vi "LEP_RV_GenerateXMLFromLinkerMapFile.vi"(9 "Linker flags":string, 10 "Compiler flags":string, 11 "Project path":path) -> ()   [LabVIEW 2011]
panel:
  out "error out":errorcluster
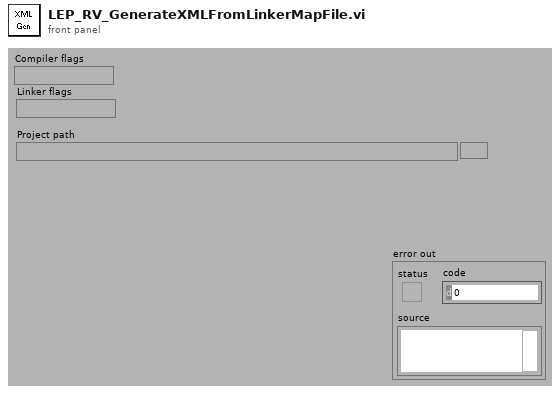
[diagram p1: front panel]
types:
  T1 = enum16{"open", "replace", "create", "open or create", "replace or create", "replace or create with confirmation"}
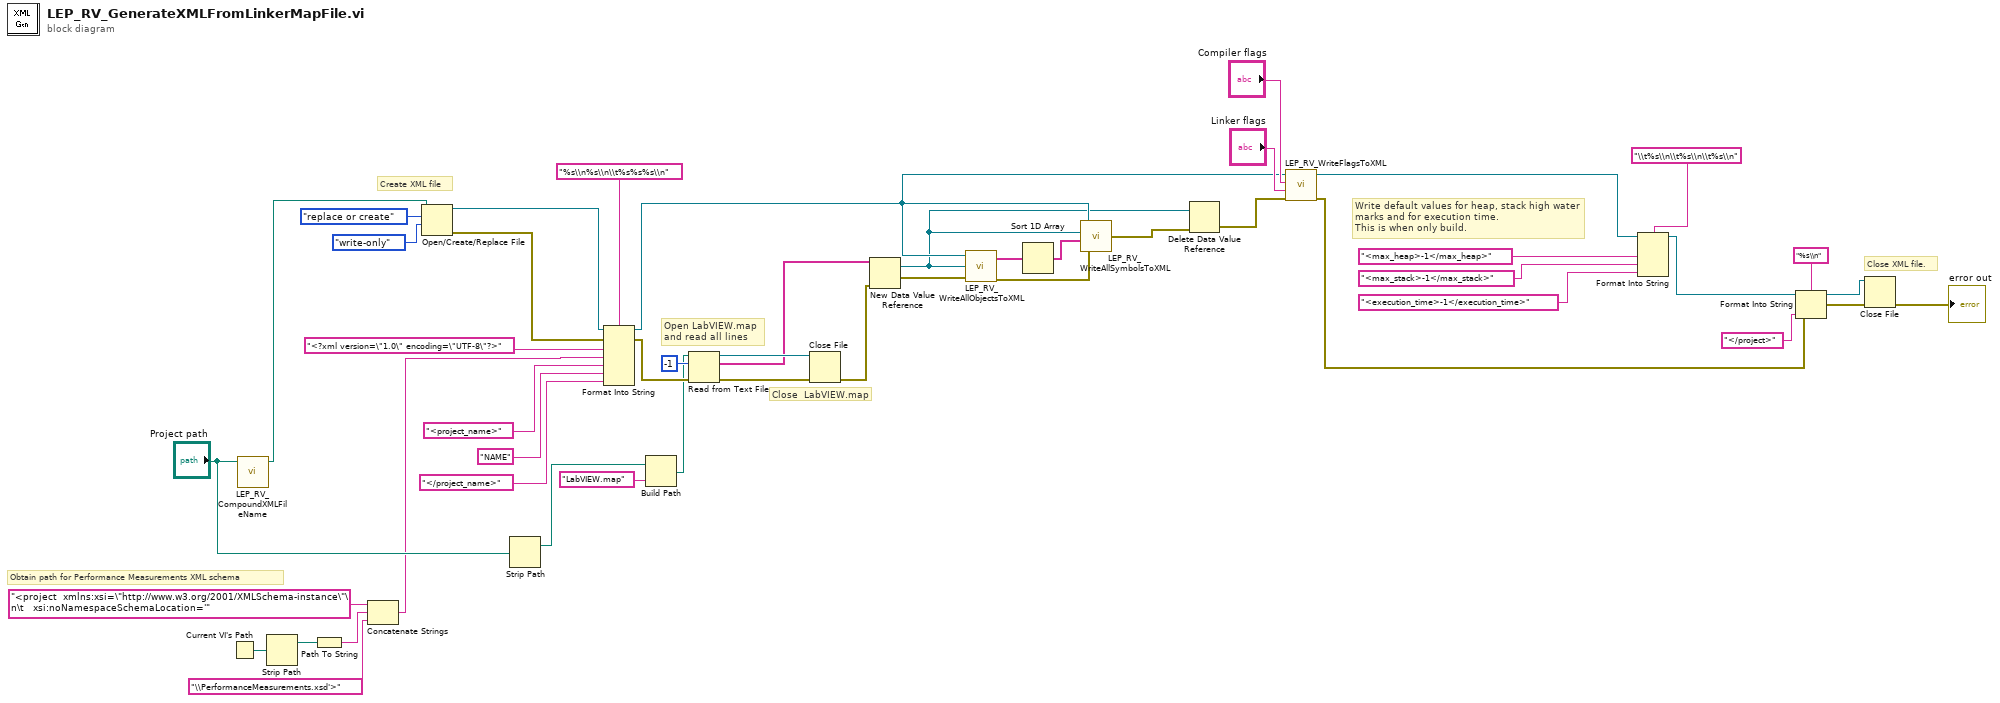
[diagram p0: block diagram]
diagram:
  # "Obtain path for Performance Measurements XML schema"
  # "Write default values for heap, stack high water marks and for execution time.\nThis is when only build."
  # "Close XML file."
  # "Close  LabVIEW.map"
  # "Open LabVIEW.map \nand read all lines"
  # "Create XML file"
  n1 = Current VI's Path() -> (path=w6:path)
  n2 = call "LEP_RV_CompoundXMLFileName.vi"("Project file path"="Project path") -> ("Path for XML generated file"=w19:path)  [unwired: 10 in]
  n3 = Strip Path(path=w6) -> (stripped path=w5:path)  [unwired: 1 out]
  n4 = Path To String(path=w5) -> (string=w3:string)
  n5 = Concatenate Strings("<project  xmlns:xsi=\"http://www.w3.org/2001/XMLSchema-instance\"\n\t   xsi:noNamespaceSchemaLocation='", w3, "\\PerformanceMeasurements.xsd'>") -> (w1:string)
  n6 = Open/Create/Replace File(file path (use dialog)=w19, operation (0:open)=T1."replace or create", access (0:read/write)=enum16{"read/write", "read-only", "write-only"}."write-only") -> (refnum out=w45:refnum<file>, error out=w44:errorcluster)  [unwired: 3 in, 1 out]
  n7 = Strip Path(path="Project path") -> (stripped path=w17:path)  [unwired: 1 out]
  n8 = Format Into String(format string="%s\\n%s\\n\\t%s%s%s\\n", initial string=w45, error in=w44, "<?xml version=\"1.0\" encoding=\"UTF-8\"?>" ("text"), w1, "<project_name>" ("input 3"), "NAME" ("input 4"), "</project_name>" ("input 5")) -> (resulting string=w21:refnum<file>, error out=w28:errorcluster)
  n9 = Build Path(base path=w17, name or relative path="LabVIEW.map") -> (appended path=w15:path)
  n10 = Read from Text File(file (use dialog)=w15, count=-1, error in=w28) -> (refnum out=w30:refnum<file>, text=w24:string[], error out=w29:errorcluster)  [unwired: 1 in, 1 out]
  n11 = Close File(refnum=w30, error in=w29) -> (error out=w23:errorcluster)  [unwired: 1 out]
  n12 = New Data Value Reference(data value=w24, error in=w23) -> (data value reference=w13:refnum<data-value>, error out=w22:errorcluster)
  n13 = call "LEP_RV_WriteAllObjectsToXML.vi"("error in"=w22, "Data value reference for\nLabVIEW.map file's lines array"=w13, "XML File Refnum"=w21) -> ("error out"=w25:errorcluster, "Array with objects' names"=w27:string[])
  n14 = Sort 1D Array(array=w27) -> (sorted array=w26:string[])
  n15 = call "LEP_RV_WriteAllSymbolsToXML.vi"("error in"=w25, "Sorted objects' names array"=w26, "Data value reference for\nLabVIEW.map file's lines array"=w13, "XML File Refnum"=w21) -> ("error out"=w14:errorcluster)
  n16 = Delete Data Value Reference(data value reference=w13, error in=w14) -> (error out=w20:errorcluster)  [unwired: 1 out]
  n17 = call "LEP_RV_WriteFlagsToXML.vi"("error in"=w20, "Linker flags"="Linker flags", "Compiler flags"="Compiler flags", "XML file refnum"=w21) -> ("error out"=w34:errorcluster, "XML file refnum"=w12:refnum<file>)  [unwired: 6 in]
  n18 = Format Into String(format string="\\t%s\\n\\t%s\\n\\t%s\\n", initial string=w12, "<max_heap>-1</max_heap>", "<max_stack>-1</max_stack>", "<execution_time>-1</execution_time>") -> (resulting string=w9:refnum<file>)  [unwired: 1 in, 1 out]
  n19 = Format Into String(format string="%s\\n", initial string=w9, error in=w34, "</project>" ("input 1")) -> (resulting string=w38:refnum<file>, error out=w35:errorcluster)
  n20 = Close File(refnum=w38, error in=w35) -> (error out=→"error out":errorcluster)  [unwired: 1 out]
